vi "Register FKs.vi"(8 "error in (no error)":errorcluster, 10 "FK/PK Info":T1, 11 "Form Model in":refnum<class "Form Model.lvclass">) -> (0 "error out":errorcluster, 3 "Form Model out":refnum<class "Form Model.lvclass">)   [LabVIEW 2020, in "Form Model.lvlib" / "Form Model.lvclass"]
uses:
  Form Model.lvclass
  C:/Program Files (x86)/National Instruments/LabVIEW 2020/vi.lib/ActorFramework/Actor/Actor.lvclass
  Forms Server/Update Fields Logic/Field FK PK Info.ctl
  <vilib>/ActorFramework/Actor/Actor.lvclass/Actor.ctl
  Form Model.lvclass/Form Model.ctl
  Forms Server/Form Server Messages Messages/Register Form FKs Msg/Register Form FKs Msg.lvclass/Register Form FKs Msg.ctl
  <vilib>/ActorFramework/Message Enqueuer/Message Enqueuer.lvclass/Message Enqueuer.ctl
  <vilib>/ActorFramework/Message Enqueuer/Enqueue.vi
  Forms Server/Form Server Messages Messages/Register Form FKs Msg/Register Form FKs Msg.lvclass
  C:/Program Files (x86)/National Instruments/LabVIEW 2020/vi.lib/ActorFramework/Message/Message.lvclass
  <vilib>/ActorFramework/Message Priority Queue/Priority Enqueue.vi
  Form Model Configuration/Form Model Configuration Class/Form Model Configuration.lvclass
  <vilib>/ActorFramework/Actor/Actor.lvclass
  Forms Server/Form Server Interfaces.lvlib
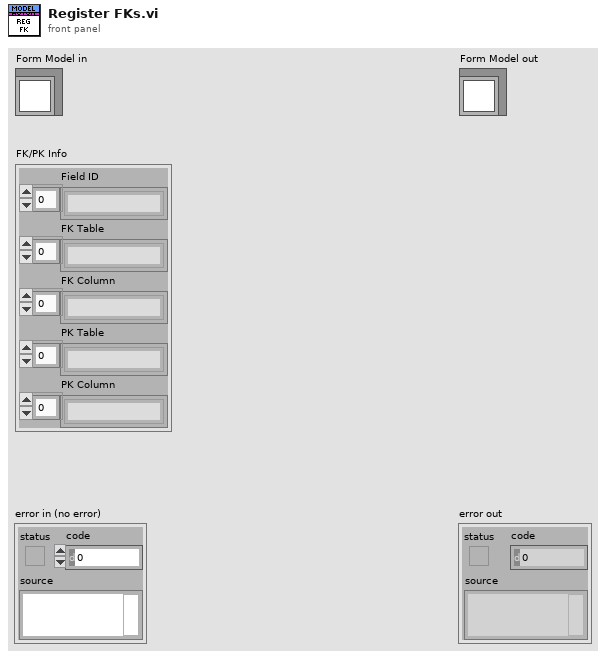
[diagram p1: front panel]
types:
  T1 = typedef "Form Server Interfaces.lvlib/Field FK PK Info.ctl" = cluster{"Field ID":string[], "FK Table":string[], "FK Column":string[], "PK Table":string[], "PK Column":string[]}
  T2 = typedef "Form Server Interfaces.lvlib/Form ID.ctl" = cluster{"Name":string, "Panel type":string}
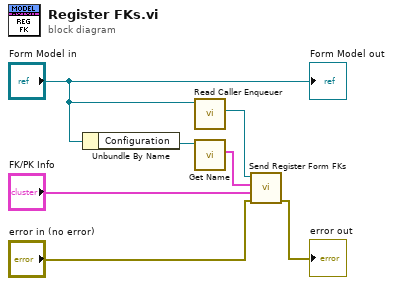
[diagram p0: block diagram]
diagram:
  n1 = Unbundle By Name("Form Model in") -> ("Configuration"=w2:refnum<class "Form Model Configuration.lvclass">)
  n2 = call <vilib>:"Read Caller Enqueuer.vi"("Actor"="Form Model in") -> ("Caller Enqueuer"=w7:refnum<class "Message Enqueuer.lvclass">)  [unwired: 10 in]
  n3 = call-dynamic "Get Name.vi"("Form Configuration in"=w2) -> ("Form ID"=w1:T2)  [unwired: 8 in, 2 out]
  n4 = call "Send Register Form FKs.vi"("error in (no error)"="error in (no error)", "FK/PK Info"="FK/PK Info", "Form ID"=w1, "Message Enqueuer"=w7) -> ("error out"=→"error out":errorcluster)  [unwired: 6 in, 1 out]
  "Form Model out" <- "Form Model in"
